vi "QA.vi"(8 "ERRIN":errorcluster caption="entrée d'erreur (pas d'erreur)") -> (0 "ERROUT":errorcluster caption="sortie d'erreur", 2 "DATAOUT":string)   [LabVIEW 2020]
uses:
  VG/VG_ATEQ.vi
panel:
  # "<\\B20\\BE:(A\\CC\\A9:P\\D2\\C5SS\\C9\\CFN\\A0HAU\\D4\\C5\\8D\\n"
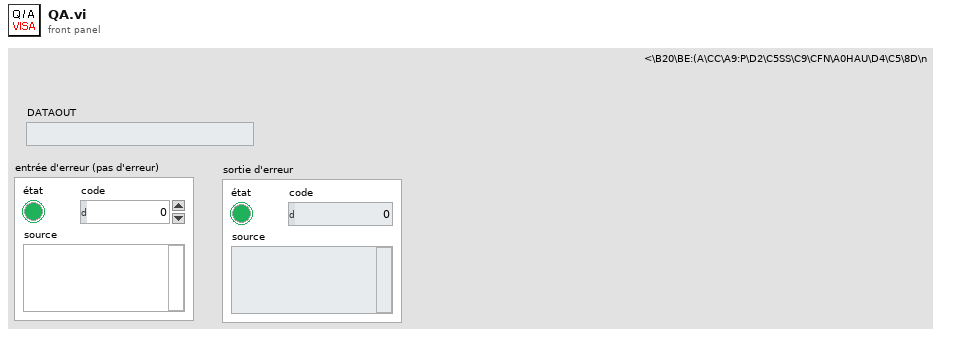
[diagram p1: front panel]
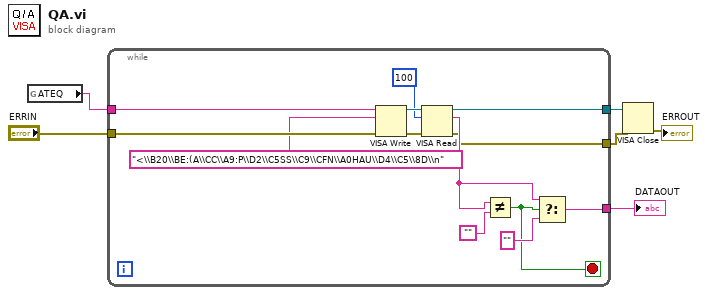
[diagram p0: block diagram]
diagram:
  n1 = global read "VG_ATEQ.vi" "ATEQ"() -> (w5:string)
  n2 = while {
    tunnel: [w19] -> w6
    tunnel: "ERRIN" -> [w12]
    tunnel: w5 -> [w11]
    tunnel: [w8] -> w3
    tunnel: [w7] -> w2
    stop <- w13 stop-if-true
    n3 = VISA Write(VISA resource name=w11, write buffer="<\\B20\\BE:(A\\CC\\A9:P\\D2\\C5SS\\C9\\CFN\\A0HAU\\D4\\C5\\8D\\n" ("buffer d'écriture"), error in (no error)=w12) -> (VISA resource name out=w17:refnum<visa-resource-name>, error out=w18:errorcluster)  [unwired: 1 out]
    n4 = VISA Read(VISA resource name=w17, byte count=u32 100 ("nombre d'octets"), error in (no error)=w18) -> (VISA resource name out=w7:refnum<visa-resource-name>, read buffer=w14:string, error out=w8:errorcluster)  [unwired: 1 out]
    n5 = Not Equal?(x=w14, y="") -> (x != y?=w13:bool)
    n6 = Select(t=w14, s=w13, f="") -> (s? t:f=w19:string)
  }
  "DATAOUT" <- w6
  n7 = VISA Close(VISA resource name=w2, error in (no error)=w3) -> (error out=→"ERROUT":errorcluster)
